vi "SpectralClustering.vi"(8 "error in":errorcluster) -> (0 "error out":errorcluster, 3 "out":refnum<class "SpectralClustering.lvclass">)   [LabVIEW 2020]
doc: "Apply clustering to a projection of the normalized Laplacian.\n\n In practice Spectral Clustering is very useful when the structure of\n the individual clusters is highly non-convex, or more generally when\n a measure of the center and spread of the cluster is not a suitable\n description of the complete cluster, such as when clusters are\n nested circles on the 2D plane.\n\n If the affinity matrix is the adjacency matrix of a graph, this method\n can be used to find normalized graph cuts.\n\n When calling ``fit``, an affinity matrix is constructed using either\n a kernel function such the Gaussian (aka RBF) kernel with Euclidean\n distance ``d(X, X)``::\n\n np.exp(-gamma * d(X,X) ** 2)\n\n or a k-nearest neighbors connectivity matrix.\n\n Alternatively, a user-provided affinity matrix can be specified by\n setting ``affinity='precomputed'``.\n\n Read more in the :ref:`User Guide <spectral_clustering>`.\n\n Parameters\n ----------\n n_clusters : int, default=8\n The dimension of the projection subspace.\n\n eigen_solver : {'arpack', 'lobpcg', 'amg'}, default=None\n The eigenvalue decomposition strategy to use. AMG requires pyamg\n to be installed. It can be faster on very large, sparse problems,\n but may also lead to instabilities. If None, then ``'arpack'`` is\n used.\n\n n_components : int, default=n_clusters\n Number of eigenvectors to use for the spectral embedding\n\n random_state : int, RandomState instance, default=None\n A pseudo random number generator used for the initialization of the\n lobpcg eigenvectors decomposition when ``eigen_solver='amg'`` and by\n the K-Means initialization. Use an int to make the randomness\n deterministic.\n See :term:`Glossary <random_state>`.\n\n n_init : int, default=10\n Number of time the k-means algorithm will be run with different\n centroid seeds. The final results will be the best output of n_init\n consecutive runs in terms of inertia. Only used if\n ``assign_labels='kmeans'``.\n\n gamma : float, default=1.0\n Kernel coefficient for rbf, poly, sigmoid, laplacian and chi2 kernels.\n Ignored for ``affinity='nearest_neighbors'``.\n\n affinity : str or callable, default='rbf'\n How to construct the affinity matrix.\n - 'nearest_neighbors': construct the affinity matrix by computing a\n graph of nearest neighbors.\n - 'rbf': construct the affinity matrix using a radial basis function\n (RBF) kernel.\n - 'precomputed': interpret ``X`` as a precomputed affinity matrix,\n where larger values indicate greater similarity between instances.\n - 'precomputed_nearest_neighbors': interpret ``X`` as a sparse graph\n of precomputed distances, and construct a binary affinity matrix\n from the ``n_neighbors`` nearest neighbors of each instance.\n - one of the kernels supported by\n :func:`~sklearn.metrics.pairwise_kernels`.\n\n Only kernels that produce similarity scores (non-negative values that\n increase with similarity) should be used. This property is not checked\n by the clustering algorithm.\n\n n_neighbors : int, default=10\n Number of neighbors to use when constructing the affinity matrix using\n the nearest neighbors method. Ignored for ``affinity='rbf'``.\n\n eigen_tol : float, default=0.0\n Stopping criterion for eigendecomposition of the Laplacian matrix\n when ``eigen_solver='arpack'``.\n\n assign_labels : {'kmeans', 'discretize'}, default='kmeans'\n The strategy for assigning labels in the embedding space. There are two\n ways to assign labels after the Laplacian embedding. k-means is a\n popular choice, but it can be sensitive to initialization.\n Discretization is another approach which is less sensitive to random\n initialization.\n\n degree : float, default=3\n Degree of the polynomial kernel. Ignored by other kernels.\n\n coef0 : float, default=1\n Zero coefficient for polynomial and sigmoid kernels.\n Ignored by other kernels.\n\n kernel_params : dict of str to any, default=None\n Parameters (keyword arguments) and values for kernel passed as\n callable object. Ignored by other kernels.\n\n n_jobs : int, default=None\n The number of parallel jobs to run when `affinity='nearest_neighbors'`\n or `affinity='precomputed_nearest_neighbors'`. The neighbors search\n will be done in parallel.\n ``None`` means 1 unless in a :obj:`joblib.parallel_backend` context.\n ``-1`` means using all processors. See :term:`Glossary <n_jobs>`\n for more details.\n\n verbose : bool, default=False\n Verbosity mode.\n\n .. versionadded:: 0.24\n\n Attributes\n ----------\n affinity_matrix_ : array-like of shape (n_samples, n_samples)\n Affinity matrix used for clustering. Available only after calling\n ``fit``.\n\n labels_ : ndarray of shape (n_samples,)\n Labels of each point\n\n \nAvailable methods:\nGet Attributes\nGet Params\nSet Params"
uses:
  SpectralClustering.lvclass
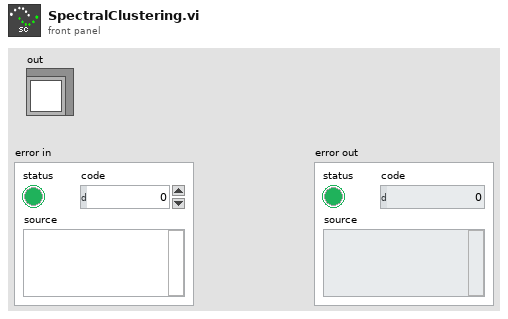
[diagram p1: front panel]
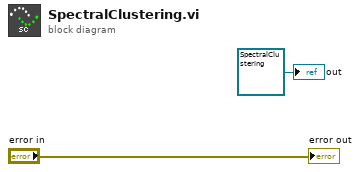
[diagram p0: block diagram]
diagram:
  "out" <- refnum<class "SpectralClustering.lvclass"> refnum ("model")
  "error out" <- "error in"
